vi "Control Intake.vi"(11 "Avoid Race Condition":bool) -> ()   [LabVIEW 2020]
uses:
  Framework/Robot Global Data.vi
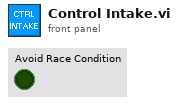
[diagram p1: front panel]
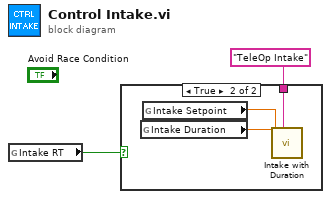
[diagram p0: block diagram]
diagram:
  n1 = global read "Robot Global Data.vi" "Intake RT"() -> (w1:bool)
  n2 = case shown="True" w1 {
    tunnel: "TeleOp Intake" ("Description") -> [_ w5]
    frame False {
    }
    frame True {
      n3 = global read "Robot Global Data.vi" "Intake Duration"() -> (w3:dbl)
      n4 = global read "Robot Global Data.vi" "Intake Setpoint"() -> (w4:dbl)
      n5 = call "Intake with Duration.vi"("Description"=w5, "Duration (s)"=w3, "Setpoint"=w4) -> ()  [unwired: 8 in, 1 out]
    }
  }
